vi "K2400 Default Set Up.vi"(8 "Error In":errorcluster, 11 "Ke2400 In":refnum<visa-resource-name>) -> (0 "Error Out":errorcluster, 3 "Ke2400 Out":refnum<visa-resource-name>)   [LabVIEW 2017]
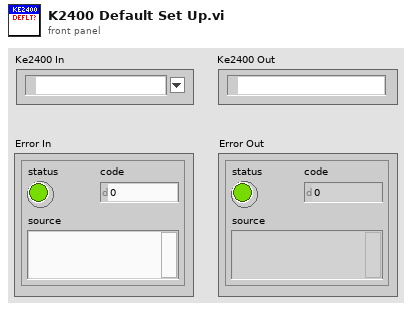
[diagram p1: front panel]
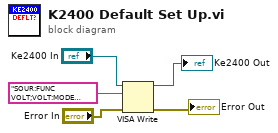
[diagram p0: block diagram]
diagram:
  n1 = VISA Write(VISA resource name="Ke2400 In", write buffer="SOUR:FUNC VOLT;VOLT:MODE FIX;RANG 100;LEV 0.0;:SENS:FUNC \"CURR\";CURR:PROT 60E-3;RANG 100E-3;:OUTP ON", error in (no error)="Error In") -> (VISA resource name out=→"Ke2400 Out":refnum<visa-resource-name>, error out=→"Error Out":errorcluster)  [unwired: 1 out]
